vi "String Byte to Norm.vi"(1 "Byte String In":string) -> (0 "String Out":string)   [LabVIEW 2025]
doc: "Author: Scott Hannahs <sth@magnet.fsu.edu>\n\nThis software is licensed for use under the “MIT License\"\nCopyright (c) 2025 Scott Hannahs, sth@sth@magnet.sthnet.net\n\nPermission is hereby granted, free of charge, to any person obtaining a copy of this software and associated documentation files (the \"Software\"), to deal in the Software without restriction, including without limitation the rights to use, copy, modify, merge, publish, distribute, sublicense, and/or sell copies of the Software, and to permit persons to whom the Software is furnished to do so, subject to the following conditions: The above copyright notice and this permission notice shall be included in all copies or substantial portions of the Software.\n\nTHE SOFTWARE IS PROVIDED \"AS IS\", WITHOUT WARRANTY OF ANY KIND, EXPRESS OR IMPLIED, INCLUDING BUT NOT LIMITED TO THE WARRANTIES OF MERCHANTABILITY, FITNESS FOR A PARTICULAR PURPOSE AND NONINFRINGEMENT. IN NO EVENT SHALL THE AUTHORS OR COPYRIGHT HOLDERS BE LIABLE FOR ANY CLAIM, DAMAGES OR OTHER LIABILITY, WHETHER IN AN ACTION OF CONTRACT, TORT OR OTHERWISE, ARISING FROM, OUT OF OR IN CONNECTION WITH THE SOFTWARE OR THE USE OR OTHER DEALINGS IN THE SOFTWARE."
panel:
  in  "delimiter":string="A"
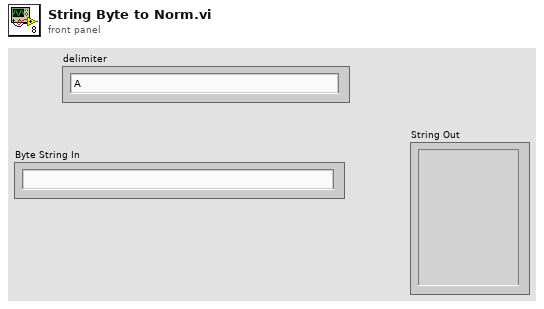
[diagram p1: front panel]
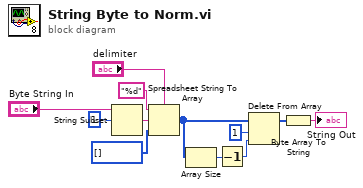
[diagram p0: block diagram]
diagram:
  n1 = String Subset(string="Byte String In", offset (0)=1) -> (substring=w2:string)  [unwired: 1 in]
  n2 = Spreadsheet String To Array(delimiter (Tab)="delimiter", format string="%d", spreadsheet string=w2, array type (2D Dbl)=u8[] [] ("unsigned byte array")) -> (array=w8:u8[])
  n3 = Array Size(array=w8) -> (size(s)=w6:i32)
  n4 = Decrement(x=w6) -> (x-1=w5:i32)
  n5 = Delete From Array(array=w8, length=1, index=w5) -> (array with subset deleted=w4:u8[])  [unwired: 1 out]
  n6 = Byte Array To String(unsigned byte array=w4) -> (string=→"String Out":string)
